vi "testUnsupportedType.vi"() -> ()   [LabVIEW 2019, in "AssertionTest.lvlib" / "AssertNotCount.lvlib"]
uses:
  AssertNotCount.lvlib
  Assertion/Assertion.lvlib
panel:
  out "error out":errorcluster
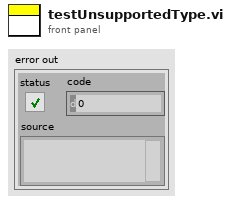
[diagram p1: front panel]
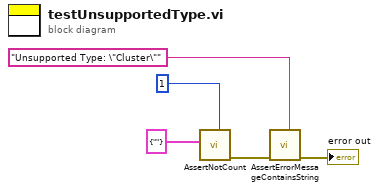
[diagram p0: block diagram]
diagram:
  n1 = call "AssertNotCount.vi"("Expected"=1, "Haystack"=cluster{string} {""}) -> ("error out"=w3:errorcluster)  [unwired: 9 in]
  n2 = call "AssertErrorMessageContainsString.vi"("Expected"="Unsupported Type: \"Cluster\"", "error in (no error)"=w3) -> ("error out"=→"error out":errorcluster)  [unwired: 9 in]
